vi "Zadanie 2.vi"() -> ()   [LabVIEW 2020]
panel:
  out "Zajêtoœæ":bool
  out "Liczby":dbl[](array[numeric])
  out "Obecnie generowana liczba":dbl
  in  "stop":bool
  out "Zliczenie producent":i32
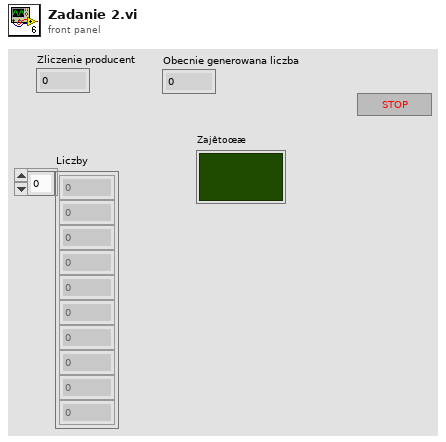
[diagram p1: front panel]
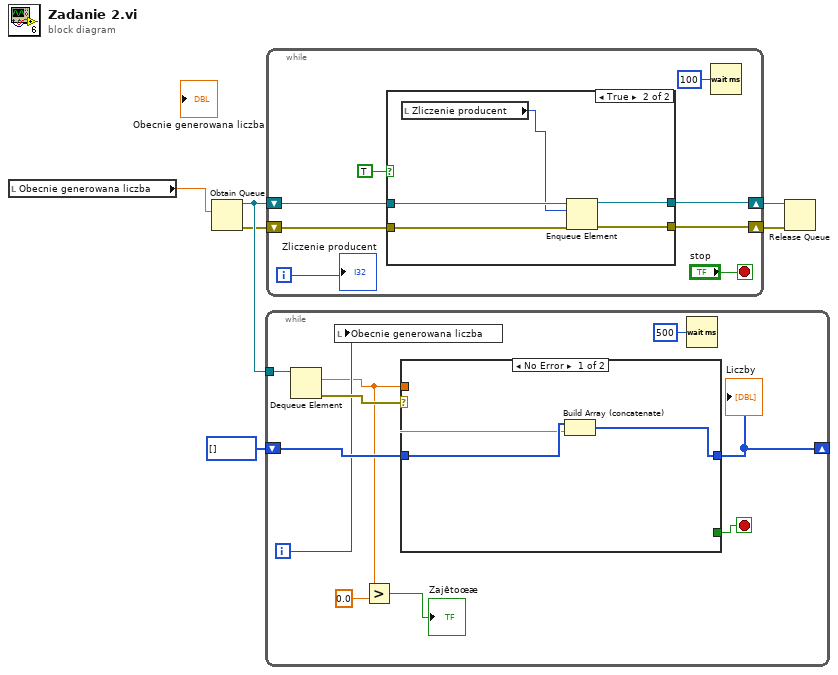
[diagram p0: block diagram]
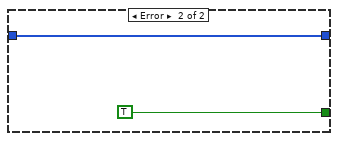
[diagram p2: hidden frame]
diagram:
  n1 = local read "Obecnie generowana liczba"() -> (w2:dbl)
  n2 = Obtain Queue(element data type=w2) -> (queue out=w6:refnum<queue>, error out=w5:errorcluster)  [unwired: 4 in, 1 out]
  n3 = while {
    tunnel: w6 -> [w16]
    shift-right: [w12] -> _
    shift-left: i32[] [] -> [w13]
    i -> [w10]
    stop <- w14 stop-if-true
    n4 = Dequeue Element(queue=w16) -> (element=w8:dbl, error out=w15:errorcluster)  [unwired: 2 in, 2 out]
    n5 = local write "Obecnie generowana liczba"(w10) -> ()
    n6 = Greater?(x=w8, y=0.0) -> (0:→"Zajêtoœæ":bool)
    n7 = case shown="No Error" w15 {
      tunnel: w8 -> [w17 _]
      tunnel: [_ TRUE] -> w14
      tunnel: [w19 w20] -> w12
      tunnel: w13 -> [w18 w20]
      frame No Error {
        n8 = Build Array (concatenate)(w18, w17) -> (w19:i32[])
      }
      frame Error {
      }
    }
    "Liczby" <- w12
    n9 = Wait (ms)(milliseconds to wait=u32 500) -> ()  [unwired: 1 out]
  }
  n10 = while {
    shift-right: [w25] -> w3
    shift-left: w5 -> [w26]
    shift-right: [w27] -> w4
    shift-left: w6 -> [w28]
    i -> [w22]
    stop <- "stop" stop-if-true
    n11 = case shown="True" TRUE ("Case Constant\n(See Context Help)") {
      tunnel: w28 -> [w31 w36]
      tunnel: [w31 w35] -> w27
      tunnel: w26 -> [w30 w34]
      tunnel: [w30 w33] -> w25
      frame False {
      }
      frame True {
        n12 = local read "Zliczenie producent"() -> (w32:i32)
        n13 = Enqueue Element(queue=w36, element=w32, error in (no error)=w34) -> (queue out=w35:refnum<queue>, error out=w33:errorcluster)  [unwired: 1 in, 1 out]
      }
    }
    n14 = Wait (ms)(milliseconds to wait=u32 100) -> ()  [unwired: 1 out]
    "Zliczenie producent" <- w22
  }
  n15 = Release Queue(queue=w4, error in (no error)=w3) -> ()  [unwired: 1 in, 3 out]
